vi "Scripting_GetAllNodesConnectedToTerminal.vi"(0 "Term Refnum":refnum<vi>, 2 "NodeTypesToFind":string[](array[string]), 3 "CreateParentTerminals(False)":bool, 5 "error in":errorcluster, 7 "StopCriteria":T1) -> (15 "Nodes":refnum<vi>[](array[refnum]), 16 "NodeTypes":string[](array[string]), 17 "ParentTerminal":refnum<vi>[](array[refnum]), 19 "error out":errorcluster)   [LabVIEW 2014]
uses:
  <resource>/Framework/Providers/Open_GDS/ClassProviders/Common/ScriptingFunctions/Scripting_FollowWireDownStreams_StopCriteria.ctl
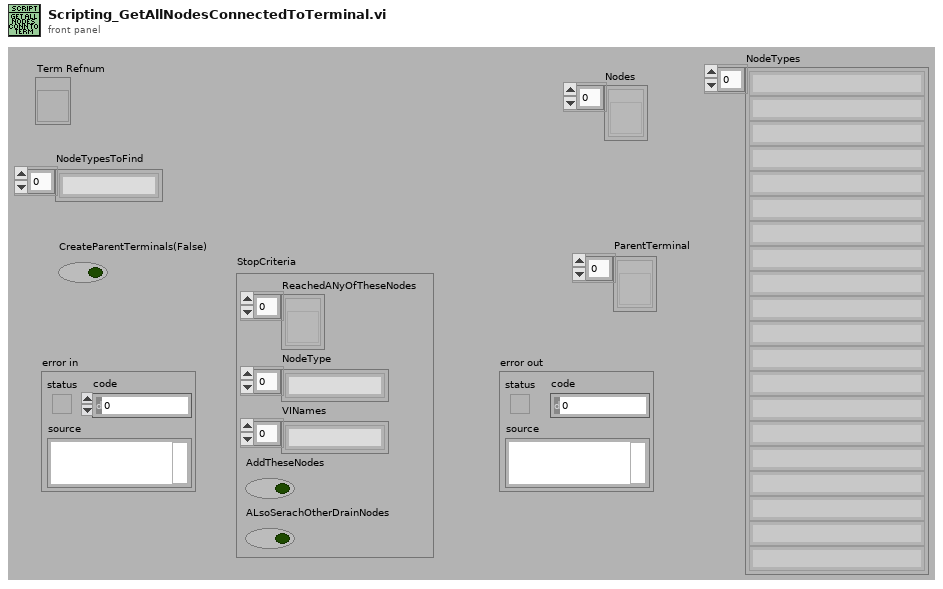
[diagram p1: front panel]
types:
  T1 = typedef "Scripting_FollowWireDownStreams_StopCriteria.ctl" = cluster{"ReachedANyOfTheseNodes":refnum<vi>[], "NodeType":string[], "VINames":string[], "AddTheseNodes":bool, "ALsoSerachOtherDrainNodes":bool}
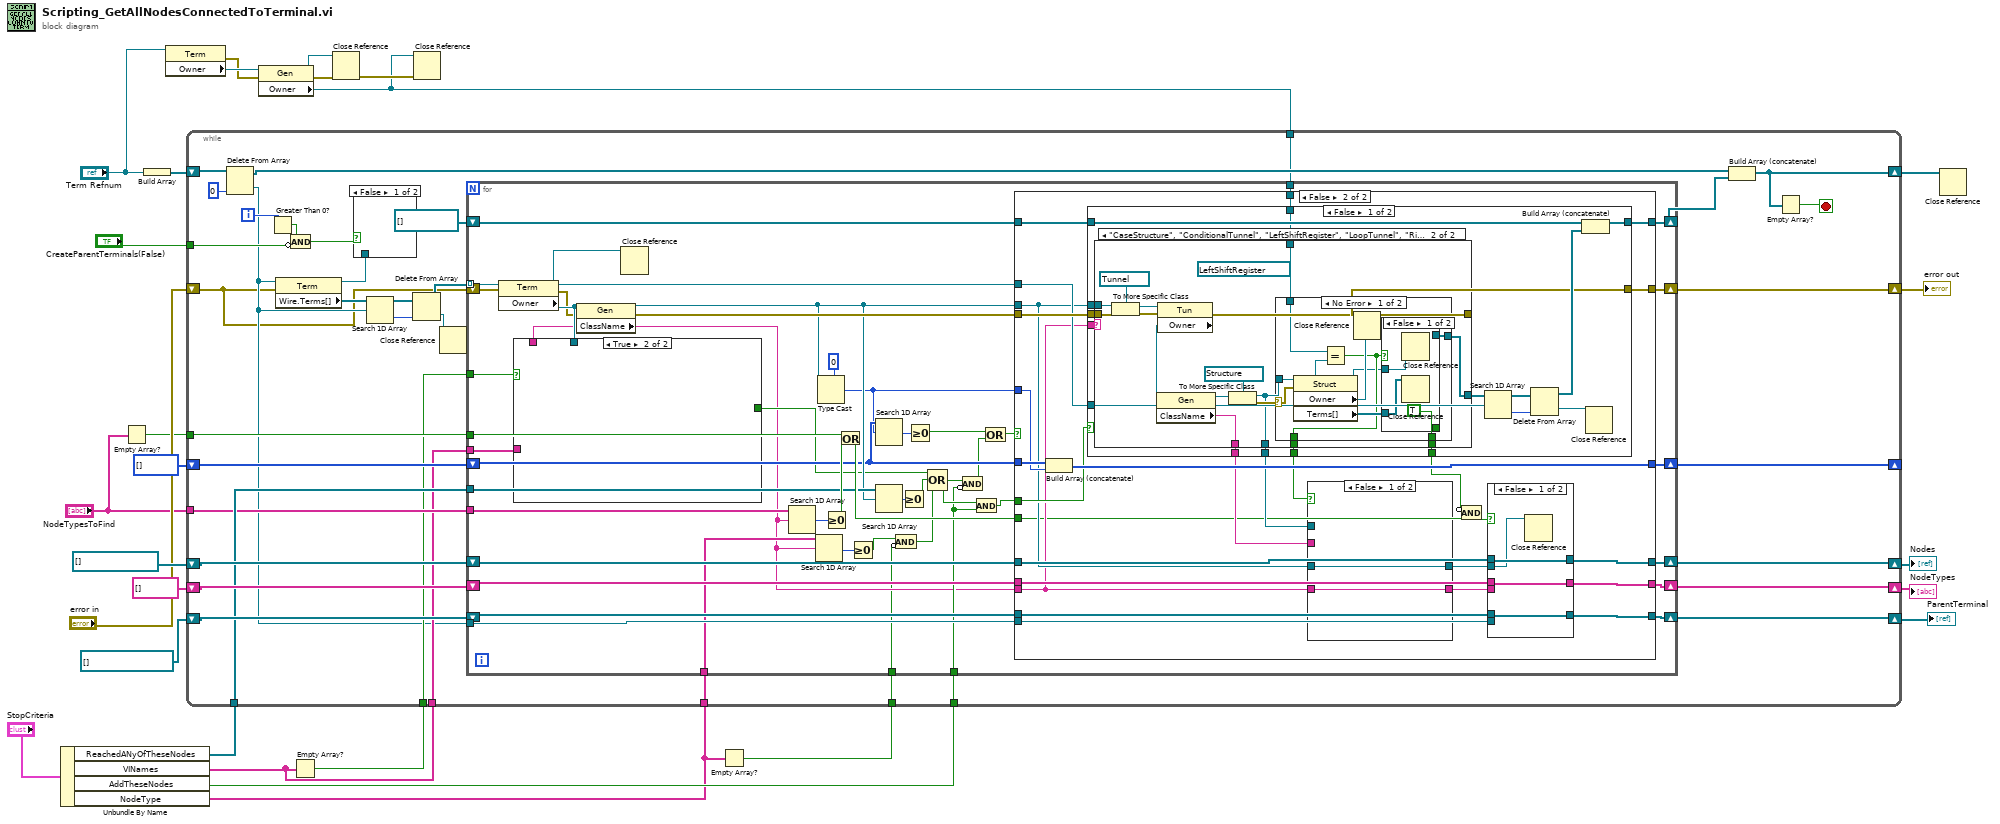
[diagram p0: block diagram]
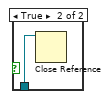
[diagram p2: hidden frame]
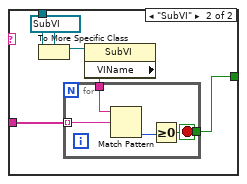
[diagram p4: hidden frame]
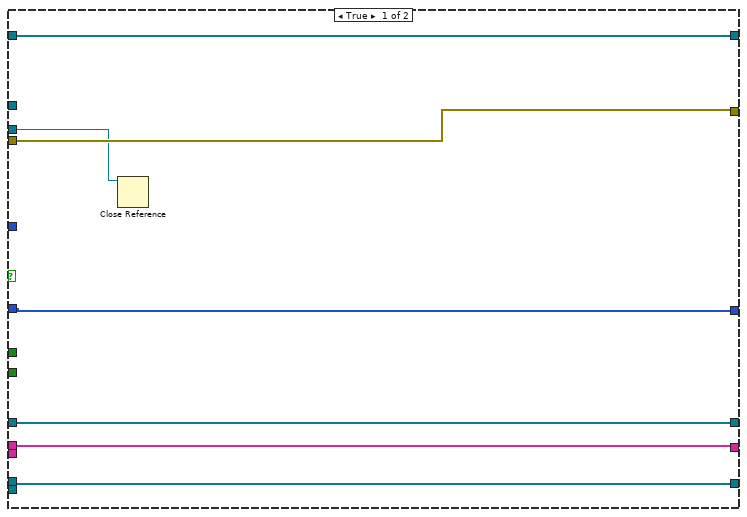
[diagram p5: hidden frame]
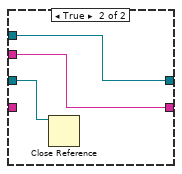
[diagram p6: hidden frame]
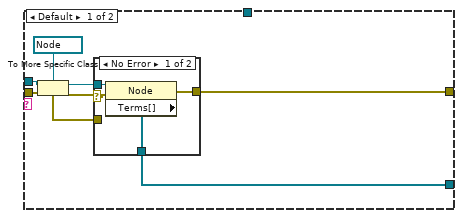
[diagram p7: hidden frame]
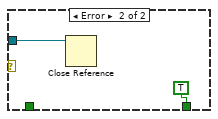
[diagram p10: hidden frame]
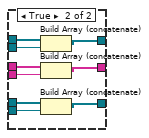
[diagram p12: hidden frame]
diagram:
  n1 = Unbundle By Name("StopCriteria") -> ("ReachedANyOfTheseNodes"=w16:refnum<vi>[], "VINames"=w11:string[], "AddTheseNodes"=w10:bool, "NodeType"=w9:string[])
  n2 = Empty Array?(array="NodeTypesToFind") -> (empty?=w13:bool)
  n3 = Build Array("Term Refnum") -> (w27:refnum<vi>[])
  n4 = property class="Term"(reference="Term Refnum") -> (error out=w5:errorcluster, "Owner"=w6:refnum<vi>)  [unwired: 1 in, 1 out]
  n5 = property class="Gen"(reference=w6, error in=w5) -> (reference out=w3:refnum<vi>, error out=w4:errorcluster, "Owner"=w1:refnum<vi>)
  n6 = Empty Array?(array=w11) -> (empty?=w12:bool)
  n7 = Close Reference(reference=w3, error in (no error)=w4) -> (error out=w2:errorcluster)
  n8 = Close Reference(reference=w1, error in (no error)=w2) -> ()  [unwired: 1 out]
  n9 = Empty Array?(array=w9) -> (empty?=w8:bool)
  n10 = while {
    shift-right: [w57] -> w28
    shift-left: w27 -> [w64]
    tunnel: "NodeTypesToFind" -> [w46]
    shift-right: [w59] -> w23
    shift-left: refnum<vi>[] [] -> [w60]
    shift-right: [w58] -> w25
    shift-left: "error in" -> [w29]
    shift-right: [w55] -> w21
    shift-left: string[] [] -> [w54]
    shift-right: [w52] -> w20
    shift-left: refnum<vi>[] [] ("ParentTerminal") -> [w53]
    tunnel: "CreateParentTerminals(False)" -> [w49]
    tunnel: w16 -> [w47]
    shift-right: [w44] -> _
    shift-left: u32[] [] -> [w45]
    tunnel: w13 -> [w42]
    tunnel: w12 -> [w41]
    tunnel: w11 -> [w40]
    tunnel: w10 -> [w39]
    tunnel: w9 -> [w32]
    tunnel: w8 -> [w31]
    tunnel: w1 -> [w30]
    i -> [w51]
    stop <- w56 stop-if-true
    n11 = Delete From Array(array=w64, index=0) -> (deleted portion=w34:refnum<vi>, array with subset deleted=w63:refnum<vi>[])  [unwired: 1 in]
    n12 = Greater Than 0?(x=w51) -> (x > 0?=w50:bool)
    n13 = property class="Term"(reference=w34, error in=w29) -> (reference out=w33:refnum<vi>, "Wire.Terms[]"=w38:refnum<vi>[])  [unwired: 1 out]
    n14 = Compound Arithmetic op=AND(w50, invert w49) -> (w48:bool)
    n15 = case shown="False" w48 {
      tunnel: w33 -> [_ w65]
      frame False {
      }
      frame True {
        n16 = Close Reference(reference=w65) -> ()  [unwired: 1 in, 1 out]
      }
    }
    n17 = Search 1D Array(1D array=w38, element=w34) -> (index of element=w37:i32)  [unwired: 1 in]
    n18 = Delete From Array(array=w38, index=w37) -> (deleted portion=w36:refnum<vi>, array with subset deleted=w35:refnum<vi>[])  [unwired: 1 in]
    n19 = Close Reference(reference=w36) -> ()  [unwired: 1 in, 1 out]
    n20 = for {
      tunnel: w35 -> [w111] mode=indexing
      tunnel: w46 -> [w97]
      shift-right: [w109] -> w59
      shift-left: w60 -> [w110]
      shift-right: [w101] -> w58
      shift-left: w29 -> [w108]
      shift-right: [w107] -> w61
      shift-left: refnum<vi>[] [] -> [w106]
      shift-right: [w104] -> w55
      shift-left: w54 -> [w103]
      shift-right: [w99] -> w52
      shift-left: w53 -> [w100]
      tunnel: w34 -> [w98]
      tunnel: w47 -> [w93]
      tunnel: w42 -> [w96]
      shift-right: [w92] -> w44
      shift-left: w45 -> [w89]
      tunnel: w41 -> [w83]
      tunnel: w40 -> [w81]
      tunnel: w39 -> [w76]
      tunnel: w32 -> [w72]
      tunnel: w31 -> [w68]
      tunnel: w30 -> [w66]
      n21 = property class="Term"(reference=w111, error in=w108) -> (reference out=w73:refnum<vi>, error out=w74:errorcluster, "Owner"=w82:refnum<vi>)
      n22 = property class="Gen"(reference=w82, error in=w74) -> (reference out=w91:refnum<vi>, error out=w102:errorcluster, "ClassName"=w71:string)
      n23 = case shown="True" w83 {
        tunnel: w71 -> [w115 _]
        tunnel: w82 -> [w114 _]
        tunnel: w81 -> [w113 _]
        tunnel: [w112 _] -> w79
        frame False {
          n24 = case shown="Default" w115 {
            tunnel: w114 -> [_ w121]
            tunnel: w113 -> [_ w117]
            tunnel: [_ w116] -> w112
            frame Default {
            }
            frame "SubVI" {
              n25 = To More Specific Class(target class=refnum<vi> refnum ("Owner"), reference=w121) -> (specific class reference=w119:refnum<vi>)  [unwired: 1 in, 1 out]
              n26 = property class="SubVI"(reference=w119) -> ("VIName"=w118:string)  [unwired: 1 in, 2 out]
              n27 = for {
                tunnel: w118 -> [w125]
                tunnel: w117 -> [w124] mode=indexing
                tunnel: [w122] -> w116
                stop <- w122 stop-if-true
                n28 = Match Pattern(string=w125, regular expression=w124) -> (offset past match=w123:i32)  [unwired: 1 in, 3 out]
                n29 = Greater Or Equal To 0?(x=w123) -> (x >= 0?=w122:bool)
              }
            }
          }
        }
        frame True {
        }
      }
      n30 = Close Reference(reference=w73) -> ()  [unwired: 1 in, 1 out]
      n31 = Search 1D Array(1D array=w97, element=w71) -> (index of element=w105:i32)  [unwired: 1 in]
      n32 = Search 1D Array(1D array=w72, element=w71) -> (index of element=w70:i32)  [unwired: 1 in]
      n33 = Type Cast(type=u32 0 ("index"), x=w91) -> (*(type *) &x=w88:u32)
      n34 = Greater Or Equal To 0?(x=w105) -> (x >= 0?=w95:bool)
      n35 = Or(x=w96, y=w95) -> (x .or. y?=w94:bool)
      n36 = Greater Or Equal To 0?(x=w70) -> (x >= 0?=w69:bool)
      n37 = Search 1D Array(1D array=w89, element=w88) -> (index of element=w86:i32)  [unwired: 1 in]
      n38 = Search 1D Array(1D array=w93, element=w91) -> (index of element=w87:i32)  [unwired: 1 in]
      n39 = Compound Arithmetic op=AND(w69, invert w68) -> (w67:bool)
      n40 = Greater Or Equal To 0?(x=w87) -> (x >= 0?=w80:bool)
      n41 = Greater Or Equal To 0?(x=w86) -> (x >= 0?=w85:bool)
      n42 = Compound Arithmetic op=OR(w79, w80, w67) -> (w77:bool)
      n43 = Compound Arithmetic op=AND(w77, invert w76) -> (w78:bool)
      n44 = Compound Arithmetic op=AND(w77, w76) -> (w75:bool)
      n45 = Compound Arithmetic op=OR(w85, w78) -> (w84:bool)
      n46 = case shown="False" w84 {
        tunnel: w110 -> [w130 w159]
        tunnel: [w130 w158] -> w109
        tunnel: [w132 w157] -> w107
        tunnel: w106 -> [w132 w156]
        tunnel: w94 -> [_ w135]
        tunnel: [w129 w155] -> w104
        tunnel: w103 -> [w129 w154]
        tunnel: w102 -> [w131 w153]
        tunnel: w71 -> [_ w140]
        tunnel: [w131 w149] -> w101
        tunnel: w100 -> [w128 w152]
        tunnel: [w128 w151] -> w99
        tunnel: w98 -> [_ w150]
        tunnel: w91 -> [w127 w142]
        tunnel: w89 -> [w126 w148]
        tunnel: [w126 w147] -> w92
        tunnel: w88 -> [_ w146]
        tunnel: w75 -> [_ w145]
        tunnel: w73 -> [_ w144]
        tunnel: w66 -> [_ w143]
        frame True {
          n47 = Close Reference(reference=w127) -> ()  [unwired: 1 in, 1 out]
        }
        frame False {
          n48 = Build Array (concatenate)(w148, w146) -> (w147:u32[])
          n49 = case shown="False" w145 {
            tunnel: [w180 w224] -> w157
            tunnel: w156 -> [w179 w224]
            tunnel: w153 -> [w178 w225]
            tunnel: w140 -> [w177 _]
            tunnel: [w170 w225] -> w149
            tunnel: w142 -> [w176 _]
            tunnel: w144 -> [w173 _]
            tunnel: w143 -> [w169 _]
            tunnel: [w168 _] -> w138
            tunnel: [w167 _] -> w137
            tunnel: [w166 _] -> w136
            tunnel: [w165 _] -> w133
            frame False {
              n50 = case shown="\"CaseStructure\", \"ConditionalTunnel\", \"LeftShiftRegister\", \"LoopTunnel\", \"RightShiftRegister\", \"SelectorTunnel\", \"Tunnel\"" w177 {
                tunnel: w178 -> [w181 w207]
                tunnel: [w184 w204] -> w170
                tunnel: w176 -> [w185 w203]
                tunnel: [w183 w202] -> w174
                tunnel: [_ w200] -> w168
                tunnel: w169 -> [_ w196]
                tunnel: [_ w195] -> w167
                tunnel: [_ w194] -> w166
                tunnel: [_ w193] -> w165
                frame Default {
                  n51 = To More Specific Class(target class=refnum<vi> refnum ("Owner"), reference=w185, error in=w181) -> (specific class reference=w186:refnum<vi>, error out=w182:errorcluster)
                  n52 = case shown="No Error" w182 {
                    selector: w182 -> [w188 _]
                    tunnel: w186 -> [w191 _]
                    tunnel: [w190 w192] -> w184
                    tunnel: [w189 _] -> w183
                    tunnel: w181 -> [_ w192]
                    frame No Error {
                      n53 = property class="Node"(reference=w191, error in=w188) -> (error out=w190:errorcluster, "Terms[]"=w189:refnum<vi>[])  [unwired: 1 out]
                    }
                    frame Error {
                    }
                  }
                }
                frame "CaseStructure", "ConditionalTunnel", "LeftShiftRegister", "LoopTunnel", "RightShiftRegister", "SelectorTunnel", "Tunnel" {
                  (unwired) refnum<vi> refnum ("reference")
                  n54 = To More Specific Class(target class=refnum<vi> refnum ("reference"), reference=w203, error in=w207) -> (specific class reference=w206:refnum<vi>, error out=w205:errorcluster)
                  n55 = property class="Tun"(reference=w206, error in=w205) -> (error out=w204:errorcluster, "Owner"=w201:refnum<vi>)  [unwired: 1 out]
                  n56 = property class="Gen"(reference=w201) -> (reference out=w199:refnum<vi>, "ClassName"=w200:string)  [unwired: 1 in, 1 out]
                  n57 = To More Specific Class(target class=refnum<vi> refnum ("reference"), reference=w199) -> (specific class reference=w195:refnum<vi>, error out=w197:errorcluster)  [unwired: 1 in]
                  n58 = case shown="No Error" w197 {
                    selector: w197 -> [w217 _]
                    tunnel: [w213 _] -> w202
                    tunnel: w195 -> [w216 w222]
                    tunnel: w196 -> [w215 _]
                    tunnel: [w211 _] -> w194
                    tunnel: [w210 TRUE] -> w193
                    frame No Error {
                      n59 = property class="Struct"(reference=w216, error in=w217) -> (reference out=w209:refnum<vi>, "Owner"=w212:refnum<vi>, "Terms[]"=w214:refnum<vi>[])  [unwired: 1 out]
                      n60 = Equal?(x=w215, y=w212) -> (x = y?=w211:bool)
                      n61 = Close Reference(reference=w212) -> ()  [unwired: 1 in, 1 out]
                      n62 = case shown="False" w211 {
                        tunnel: w214 -> [w220 w221]
                        tunnel: [_ w221] -> w213
                        tunnel: [TRUE _] -> w210
                        tunnel: w209 -> [w218 _]
                        frame False {
                          n63 = Close Reference(reference=w218) -> ()  [unwired: 1 in, 1 out]
                          n64 = Close Reference(reference=w220) -> ()  [unwired: 1 in, 1 out]
                        }
                        frame True {
                        }
                      }
                    }
                    frame Error {
                      n65 = Close Reference(reference=w222) -> ()  [unwired: 1 in, 1 out]
                    }
                  }
                }
              }
              n66 = Search 1D Array(1D array=w174, element=w173) -> (index of element=w175:i32)  [unwired: 1 in]
              n67 = Delete From Array(array=w174, index=w175) -> (deleted portion=w172:refnum<vi>, array with subset deleted=w171:refnum<vi>[])  [unwired: 1 in]
              n68 = Build Array (concatenate)(w179, w171) -> (w180:refnum<vi>[])
              n69 = Close Reference(reference=w172) -> ()  [unwired: 1 in, 1 out]
            }
            frame True {
            }
          }
          n70 = case shown="False" w136 {
            tunnel: w142 -> [w161 w162]
            tunnel: [w161 w163] -> w141
            tunnel: w140 -> [w160 _]
            tunnel: [w160 w164] -> w139
            tunnel: w138 -> [_ w164]
            tunnel: w137 -> [_ w163]
            frame False {
            }
            frame True {
              n71 = Close Reference(reference=w162) -> ()  [unwired: 1 in, 1 out]
            }
          }
          n72 = Compound Arithmetic op=AND(invert w133, w135) -> (w134:bool)
          n73 = case shown="False" w134 {
            tunnel: w159 -> [w229 w238]
            tunnel: [w229 w237] -> w158
            tunnel: w139 -> [_ w234]
            tunnel: w154 -> [w228 w235]
            tunnel: [w228 w236] -> w155
            tunnel: w141 -> [w227 w233]
            tunnel: w150 -> [_ w232]
            tunnel: w152 -> [w226 w231]
            tunnel: [w226 w230] -> w151
            frame False {
              n74 = Close Reference(reference=w227) -> ()  [unwired: 1 in, 1 out]
            }
            frame True {
              n75 = Build Array (concatenate)(w238, w233) -> (w237:refnum<vi>[])
              n76 = Build Array (concatenate)(w235, w234) -> (w236:string[])
              n77 = Build Array (concatenate)(w231, w232) -> (w230:refnum<vi>[])
            }
          }
        }
      }
    }
    n78 = Build Array (concatenate)(w63, w61) -> (w57:refnum<vi>[])
    n79 = Empty Array?(array=w57) -> (empty?=w56:bool)
  }
  "error out" <- w25
  "Nodes" <- w23
  "NodeTypes" <- w21
  "ParentTerminal" <- w20
  n80 = Close Reference(reference=w28) -> ()  [unwired: 1 in, 1 out]
